vi "Set Device Bit Mode.vi"(8 "error in (no error)":errorcluster, 9 "Bit Mode":u8(ring) items=["Reset Bit Mode"=0, "Asynchronous Bit Bang"=1, "MPSSE"=2, "Synchronous Bit Bang"=4, "MCU Host Bus Emulation"=8, "Fast Opto-Isolated Serial"=16, "CBUS Bit Bang"=32, "Single Channel 245 Synchronous FIFO"=64], 10 "Bit Mode Mask":u8 format="%x", 11 "Handle":u64) -> (0 "error out":errorcluster, 3 "Handle out":u64)   [LabVIEW 2019, in "D2XX-lv.lvlib"]
doc: "This function sets the device bit mode for an open device."
uses:
  D2XX-lv.lvlib
  <instrlib>/_D2XX/D2XX/D2XX.lvlib
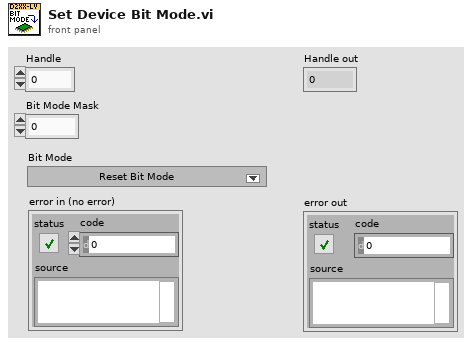
[diagram p1: front panel]
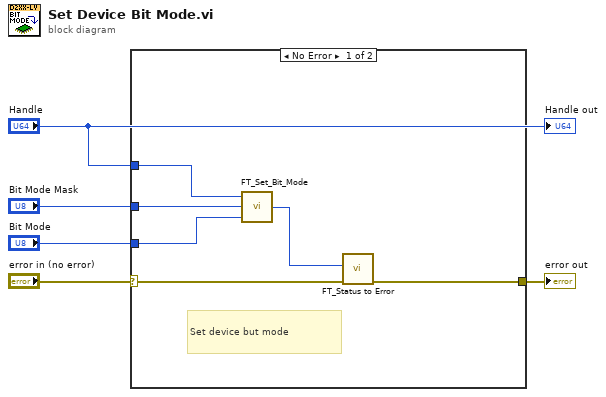
[diagram p0: block diagram]
diagram:
  n1 = case shown="No Error" "error in (no error)" {
    selector: "error in (no error)" -> [w11 w12]
    tunnel: [w8 w12] -> w4
    tunnel: "Handle" -> [w9 _]
    tunnel: "Bit Mode" -> [w7 _]
    tunnel: "Bit Mode Mask" -> [w6 _]
    frame No Error {
      # "Set device but mode"
      n2 = call <instrlib>:"FT_Set_Bit_Mode.vi"("Bit Mode"=w7, "Bit Mode Mask"=w6, "Handle"=w9) -> ("FT_Status"=w10:u32)
      n3 = call "FT_Status to Error.vi"("error in (no error)"=w11, "FT_Status"=w10) -> ("error out"=w8:errorcluster)  [unwired: 9 in]
    }
    frame Error {
    }
  }
  "error out" <- w4
  "Handle out" <- "Handle"
